vi "Update.vi"(8 "error in (no error)":errorcluster, 10 "Message in":refnum<class "UpdateMessage.lvclass">, 11 "Thorcam in":refnum<class "Thorcam.lvclass">) -> (0 "error out":errorcluster, 3 "Thorcam out":refnum<class "Thorcam.lvclass">)   [LabVIEW 2012, in "Thorcam.lvclass"]
doc: "The update method processes the command 'update'. \n\nThe command 'update' is used for receiving new values to be set to the private data of the class. This could be seen as a public set method for setting new parameters to the private class data."
uses:
  Thorcam.lvclass
  <vilib>/Distrio/Murmex/UpdateMessage/UpdateMessage.lvclass
  Thorcam.lvclass/Thorcam.ctl
  feed.ctl
  <vilib>/Distrio/Murmex/Murmex/Murmex.lvclass
panel:
  # "This method is called when the UPDATE\ntrigger is sent. \n\nOverride this method when your component needs to\nrespond to this trigger. \n\nCall parent for proper implementation"
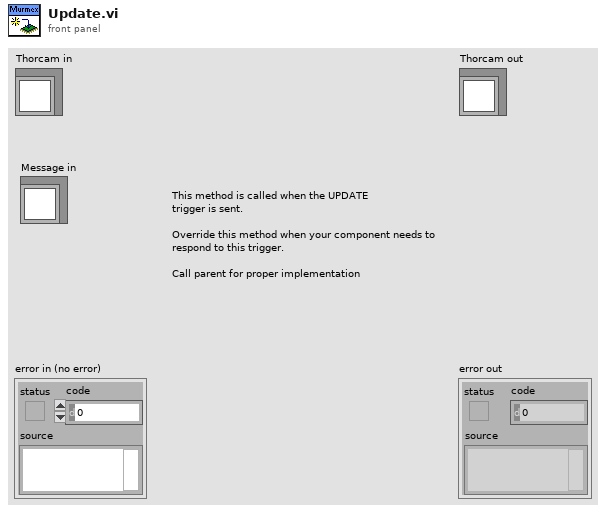
[diagram p1: front panel]
types:
  T1 = typedef "Thorcam.lvclass/feed.ctl" = enum16{"Video", "Cross Correlation", "Rob and Roy", "Roy", "Rob"}
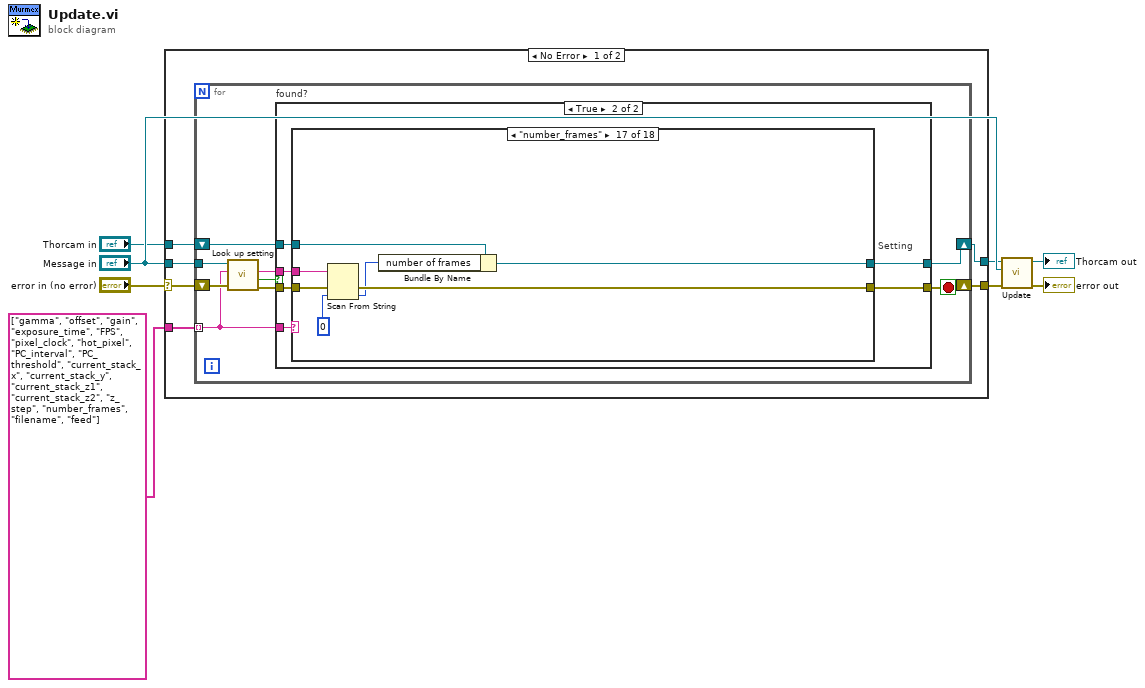
[diagram p0: block diagram]
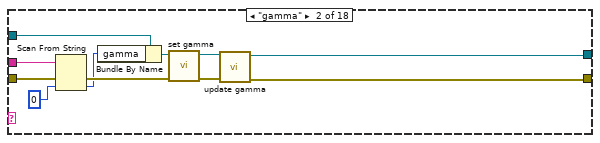
[diagram p4: hidden frame]
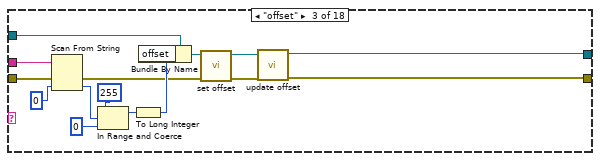
[diagram p5: hidden frame]
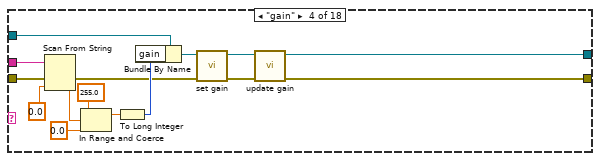
[diagram p6: hidden frame]
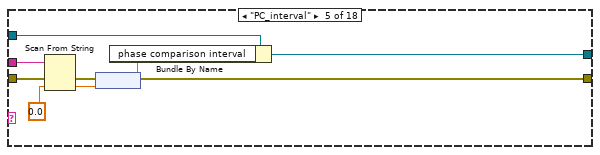
[diagram p7: hidden frame]
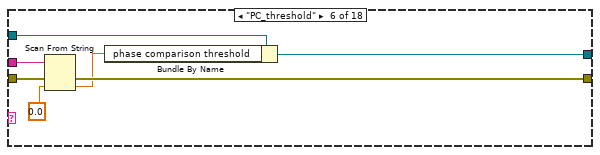
[diagram p8: hidden frame]
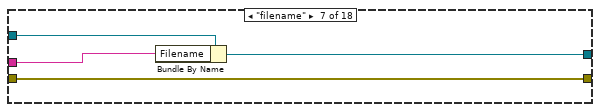
[diagram p9: hidden frame]
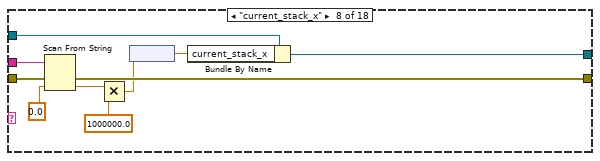
[diagram p10: hidden frame]
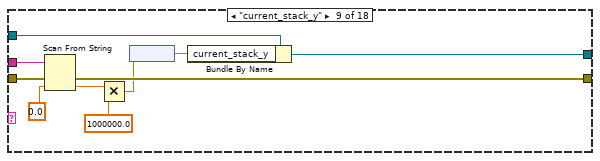
[diagram p11: hidden frame]
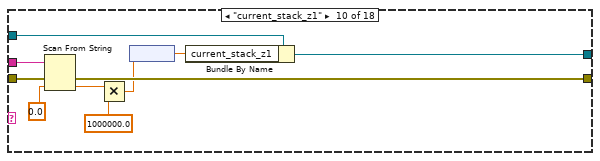
[diagram p12: hidden frame]
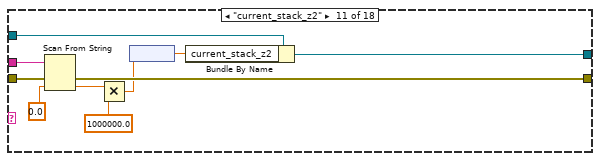
[diagram p13: hidden frame]
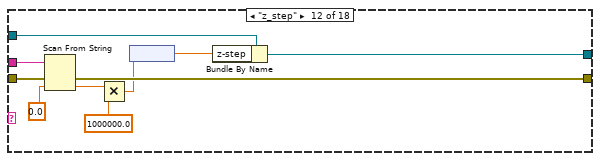
[diagram p14: hidden frame]
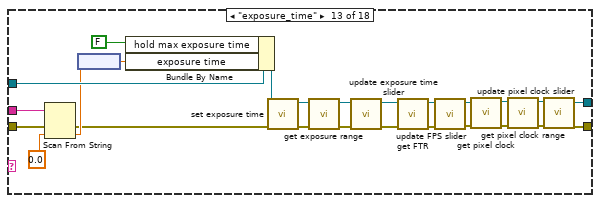
[diagram p15: hidden frame]
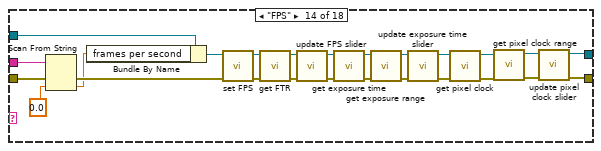
[diagram p16: hidden frame]
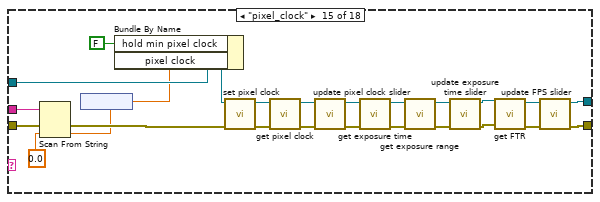
[diagram p17: hidden frame]
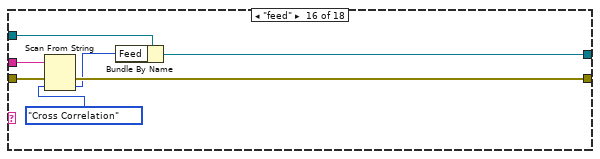
[diagram p18: hidden frame]
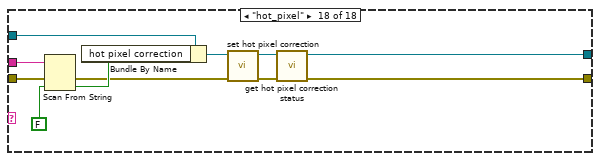
[diagram p19: hidden frame]
diagram:
  n1 = case shown="No Error" "error in (no error)" {
    selector: "error in (no error)" -> [w14 w245]
    tunnel: string[] ["gamma", "offset", "gain", "exposure_time", "FPS", "pixel_clock", "hot_pixel", "PC_interval", "PC_threshold", "current_stack_x", "current_stack_y", "current_stack_z1", "current_stack_z2", "z_step", "number_frames", "filename", "feed"] ("key chains") -> [w13 _]
    tunnel: "Message in" -> [w12 _]
    tunnel: "Thorcam in" -> [w11 w244]
    tunnel: [w10 w244] -> w2
    tunnel: [w9 w245] -> w1
    frame No Error {
      n2 = for {
        shift-right: [w16] -> w9
        shift-left: w14 -> [w23]
        tunnel: w13 -> [w21] mode=indexing
        tunnel: w12 -> [w20]
        shift-right: [w15] -> w10
        shift-left: w11 -> [w19]
        stop <- w16 stop-if-true
        n3 = call <vilib>:"Look up setting.vi"("error in (no error)"=w23, "tag name"=w21, "UpdateMessage in"=w20) -> ("error out"=w22:errorcluster, "found?"=w18:bool, "value"=w17:string)  [unwired: 5 in, 1 out]
        n4 = case "found?" shown="True" w18 {
          tunnel: w19 -> [w25 w30]
          tunnel: w17 -> [_ w31]
          tunnel: w22 -> [w24 w29]
          tunnel: w21 -> [_ w26]
          tunnel: [w25 w28] -> w15
          tunnel: [w24 w27] -> w16
          frame False {
          }
          frame True {
            n5 = case "Setting" shown="\"number_frames\"" w26 {
              tunnel: w31 -> [_ w43 w52 w73 w81 w88 w92 w102 w112 w122 w132 w142 w167 w192 w202 w224 w231 w242]
              tunnel: w30 -> [w33 w42 w59 w72 w80 w87 w93 w101 w111 w121 w131 w141 w166 w191 w218 w223 w230 w241]
              tunnel: w29 -> [w32 w44 w58 w74 w82 w89 w90 w103 w113 w123 w133 w143 w168 w193 w205 w225 w232 w243]
              tunnel: [w33 w35 w46 w60 w79 w86 w91 w100 w110 w120 w130 w140 w148 w174 w211 w222 w229 w233] -> w28
              tunnel: [w32 w34 w45 w61 w78 w85 w90 w99 w109 w119 w129 w139 w147 w170 w214 w221 w228 w236] -> w27
              frame Default {
              }
              frame "gamma" {
                n6 = Scan From String(input string=w43, error in=w44, default 1=0 ("settings.image.gamma")) -> (error out=w41:errorcluster, output 1=w39:i32)  [unwired: 2 in, 2 out]
                n7 = Bundle By Name(cluster=w42, "gamma"=w39) -> (w40:refnum<class "Thorcam.lvclass">)
                n8 = call-dynamic "set gamma.vi"("error in (no error)"=w41, "Thorcam in"=w40) -> ("error out"=w36:errorcluster, "Thorcam out"=w37:refnum<class "Thorcam.lvclass">)  [unwired: 8 in]
                n9 = call-dynamic "update gamma.vi"("error in (no error)"=w36, "Thorcam in"=w37) -> ("error out"=w34:errorcluster, "Thorcam out"=w35:refnum<class "Thorcam.lvclass">)  [unwired: 8 in]
              }
              frame "offset" {
                n10 = Scan From String(input string=w52, error in=w58, default 1=0 ("default value 1")) -> (error out=w51:errorcluster, output 1=w55:i32)  [unwired: 2 in, 2 out]
                n11 = In Range and Coerce(upper limit=255, x=w55, lower limit=0) -> (coerced(x)=w54:i32)  [unwired: 1 out]
                n12 = To Long Integer(number=w54) -> (32bit integer=w53:i32)
                n13 = Bundle By Name(cluster=w59, "offset"=w53) -> (w50:refnum<class "Thorcam.lvclass">)
                n14 = call-dynamic "set offset.vi"("error in (no error)"=w51, "Thorcam in"=w50) -> ("error out"=w47:errorcluster, "Thorcam out"=w48:refnum<class "Thorcam.lvclass">)  [unwired: 8 in]
                n15 = call-dynamic "update offset.vi"("error in (no error)"=w47, "Thorcam in"=w48) -> ("error out"=w45:errorcluster, "Thorcam out"=w46:refnum<class "Thorcam.lvclass">)  [unwired: 8 in]
              }
              frame "gain" {
                n16 = Scan From String(input string=w73, error in=w74, default 1=0.0 ("settings.Superactuator")) -> (error out=w65:errorcluster, output 1=w68:dbl)  [unwired: 2 in, 2 out]
                n17 = In Range and Coerce(upper limit=255.0, x=w68, lower limit=0.0) -> (coerced(x)=w66:dbl)  [unwired: 1 out]
                n18 = To Long Integer(number=w66) -> (32bit integer=w67:i32)
                n19 = Bundle By Name(cluster=w72, "gain"=w67) -> (w64:refnum<class "Thorcam.lvclass">)
                n20 = call-dynamic "set gain.vi"("error in (no error)"=w65, "Thorcam in"=w64) -> ("error out"=w62:errorcluster, "Thorcam out"=w63:refnum<class "Thorcam.lvclass">)  [unwired: 8 in]
                n21 = call-dynamic "update gain.vi"("error in (no error)"=w62, "Thorcam in"=w63) -> ("error out"=w61:errorcluster, "Thorcam out"=w60:refnum<class "Thorcam.lvclass">)  [unwired: 8 in]
              }
              frame "PC_interval" {
                n22 = Scan From String(input string=w81, error in=w82, default 1=0.0 ("settings.Superactuator")) -> (error out=w78:errorcluster, output 1=w76:dbl)  [unwired: 2 in, 2 out]
                n23 = node(w76) -> (w75:dbl[unit])
                n24 = Bundle By Name(cluster=w80, "phase comparison interval"=w75) -> (w79:refnum<class "Thorcam.lvclass">)
              }
              frame "PC_threshold" {
                n25 = Scan From String(input string=w88, error in=w89, default 1=0.0 ("settings.Superactuator")) -> (error out=w85:errorcluster, output 1=w83:dbl)  [unwired: 2 in, 2 out]
                n26 = Bundle By Name(cluster=w87, "phase comparison threshold"=w83) -> (w86:refnum<class "Thorcam.lvclass">)
              }
              frame "filename" {
                n27 = Bundle By Name(cluster=w93, "Filename"=w92) -> (w91:refnum<class "Thorcam.lvclass">)
              }
              frame "current_stack_x" {
                n28 = Scan From String(input string=w102, error in=w103, default 1=0.0 ("settings.Superactuator")) -> (error out=w99:errorcluster, output 1=w96:dbl)  [unwired: 2 in, 2 out]
                n29 = Multiply(x=w96, y=1000000.0) -> (x*y=w95:dbl)
                n30 = node(w95) -> (w94:dbl[unit])
                n31 = Bundle By Name(cluster=w101, "current_stack_x"=w94) -> (w100:refnum<class "Thorcam.lvclass">)
              }
              frame "current_stack_y" {
                n32 = Scan From String(input string=w112, error in=w113, default 1=0.0 ("settings.Superactuator")) -> (error out=w109:errorcluster, output 1=w106:dbl)  [unwired: 2 in, 2 out]
                n33 = Multiply(x=w106, y=1000000.0) -> (x*y=w105:dbl)
                n34 = node(w105) -> (w104:dbl[unit])
                n35 = Bundle By Name(cluster=w111, "current_stack_y"=w104) -> (w110:refnum<class "Thorcam.lvclass">)
              }
              frame "current_stack_z1" {
                n36 = Scan From String(input string=w122, error in=w123, default 1=0.0 ("settings.Superactuator")) -> (error out=w119:errorcluster, output 1=w116:dbl)  [unwired: 2 in, 2 out]
                n37 = Multiply(x=w116, y=1000000.0) -> (x*y=w115:dbl)
                n38 = node(w115) -> (w114:dbl[unit])
                n39 = Bundle By Name(cluster=w121, "current_stack_z1"=w114) -> (w120:refnum<class "Thorcam.lvclass">)
              }
              frame "current_stack_z2" {
                n40 = Scan From String(input string=w132, error in=w133, default 1=0.0 ("settings.Superactuator")) -> (error out=w129:errorcluster, output 1=w126:dbl)  [unwired: 2 in, 2 out]
                n41 = Multiply(x=w126, y=1000000.0) -> (x*y=w125:dbl)
                n42 = node(w125) -> (w124:dbl[unit])
                n43 = Bundle By Name(cluster=w131, "current_stack_z2"=w124) -> (w130:refnum<class "Thorcam.lvclass">)
              }
              frame "z_step" {
                n44 = Scan From String(input string=w142, error in=w143, default 1=0.0 ("settings.Superactuator")) -> (error out=w139:errorcluster, output 1=w136:dbl)  [unwired: 2 in, 2 out]
                n45 = Multiply(x=w136, y=1000000.0) -> (x*y=w135:dbl)
                n46 = node(w135) -> (w134:dbl[unit])
                n47 = Bundle By Name(cluster=w141, "z-step"=w134) -> (w140:refnum<class "Thorcam.lvclass">)
              }
              frame "exposure_time" {
                n48 = Scan From String(input string=w167, error in=w168, default 1=0.0 ("settings.Superactuator")) -> (error out=w160:errorcluster, output 1=w164:dbl)  [unwired: 2 in, 2 out]
                n49 = node(w164) -> (w163:dbl[unit])
                n50 = Bundle By Name(cluster=w166, "hold max exposure time"=FALSE ("runtime.exposure range.max exposure time"), "exposure time"=w163) -> (w159:refnum<class "Thorcam.lvclass">)
                n51 = call-dynamic "set exposure time.vi"("error in (no error)"=w160, "Thorcam in"=w159) -> ("error out"=w156:errorcluster, "Thorcam out"=w158:refnum<class "Thorcam.lvclass">)  [unwired: 8 in]
                n52 = call-dynamic "get exposure range.vi"("error in (no error)"=w156, "Thorcam in"=w158) -> ("error out"=w155:errorcluster, "Thorcam out"=w157:refnum<class "Thorcam.lvclass">)  [unwired: 8 in]
                n53 = call-dynamic "update exposure time slider.vi"("error in (no error)"=w155, "Thorcam in"=w157) -> ("error out"=w145:errorcluster, "Thorcam out"=w146:refnum<class "Thorcam.lvclass">)  [unwired: 8 in]
                n54 = call-dynamic "get FTR.vi"("error in (no error)"=w145, "Thorcam in"=w146) -> ("error out"=w162:errorcluster, "Thorcam out"=w161:refnum<class "Thorcam.lvclass">)  [unwired: 8 in]
                n55 = call-dynamic "update FPS slider.vi"("error in (no error)"=w162, "Thorcam in"=w161) -> ("error out"=w154:errorcluster, "Thorcam out"=w153:refnum<class "Thorcam.lvclass">)  [unwired: 8 in]
                n56 = call-dynamic "get pixel clock.vi"("error in (no error)"=w154, "Thorcam in"=w153) -> ("error out"=w151:errorcluster, "Thorcam out"=w152:refnum<class "Thorcam.lvclass">)  [unwired: 8 in]
                n57 = call-dynamic "get pixel clock range.vi"("error in (no error)"=w151, "Thorcam in"=w152) -> ("error out"=w149:errorcluster, "Thorcam out"=w150:refnum<class "Thorcam.lvclass">)  [unwired: 8 in]
                n58 = call-dynamic "update pixel clock slider.vi"("error in (no error)"=w149, "Thorcam in"=w150) -> ("error out"=w147:errorcluster, "Thorcam out"=w148:refnum<class "Thorcam.lvclass">)  [unwired: 8 in]
              }
              frame "FPS" {
                n59 = Scan From String(input string=w192, error in=w193, default 1=0.0 ("settings.Superactuator")) -> (error out=w187:errorcluster, output 1=w169:dbl)  [unwired: 2 in, 2 out]
                n60 = Bundle By Name(cluster=w191, "frames per second"=w169) -> (w186:refnum<class "Thorcam.lvclass">)
                n61 = call-dynamic "set FPS.vi"("error in (no error)"=w187, "Thorcam in"=w186) -> ("error out"=w184:errorcluster, "Thorcam out"=w185:refnum<class "Thorcam.lvclass">)  [unwired: 8 in]
                n62 = call-dynamic "get FTR.vi"("error in (no error)"=w184, "Thorcam in"=w185) -> ("error out"=w182:errorcluster, "Thorcam out"=w183:refnum<class "Thorcam.lvclass">)  [unwired: 8 in]
                n63 = call-dynamic "update FPS slider.vi"("error in (no error)"=w182, "Thorcam in"=w183) -> ("error out"=w179:errorcluster, "Thorcam out"=w181:refnum<class "Thorcam.lvclass">)  [unwired: 8 in]
                n64 = call-dynamic "get exposure time.vi"("error in (no error)"=w179, "Thorcam in"=w181) -> ("error out"=w178:errorcluster, "Thorcam out"=w180:refnum<class "Thorcam.lvclass">)  [unwired: 7 in, 1 out]
                n65 = call-dynamic "get exposure range.vi"("error in (no error)"=w178, "Thorcam in"=w180) -> ("error out"=w189:errorcluster, "Thorcam out"=w188:refnum<class "Thorcam.lvclass">)  [unwired: 8 in]
                n66 = call-dynamic "update exposure time slider.vi"("error in (no error)"=w189, "Thorcam in"=w188) -> ("error out"=w173:errorcluster, "Thorcam out"=w177:refnum<class "Thorcam.lvclass">)  [unwired: 8 in]
                n67 = call-dynamic "get pixel clock.vi"("error in (no error)"=w173, "Thorcam in"=w177) -> ("error out"=w172:errorcluster, "Thorcam out"=w176:refnum<class "Thorcam.lvclass">)  [unwired: 8 in]
                n68 = call-dynamic "get pixel clock range.vi"("error in (no error)"=w172, "Thorcam in"=w176) -> ("error out"=w171:errorcluster, "Thorcam out"=w175:refnum<class "Thorcam.lvclass">)  [unwired: 8 in]
                n69 = call-dynamic "update pixel clock slider.vi"("error in (no error)"=w171, "Thorcam in"=w175) -> ("error out"=w170:errorcluster, "Thorcam out"=w174:refnum<class "Thorcam.lvclass">)  [unwired: 8 in]
              }
              frame "pixel_clock" {
                n70 = Scan From String(input string=w202, error in=w205, default 1=0.0 ("settings.Superactuator")) -> (error out=w204:errorcluster, output 1=w203:dbl)  [unwired: 2 in, 2 out]
                n71 = node(w203) -> (w217:dbl[unit])
                n72 = Bundle By Name(cluster=w218, "hold min pixel clock"=FALSE ("runtime.pixel clock range.hold minimum"), "pixel clock"=w217) -> (w210:refnum<class "Thorcam.lvclass">)
                n73 = call-dynamic "set pixel clock.vi"("error in (no error)"=w204, "Thorcam in"=w210) -> ("error out"=w196:errorcluster, "Thorcam out"=w198:refnum<class "Thorcam.lvclass">)  [unwired: 8 in]
                n74 = call-dynamic "get pixel clock.vi"("error in (no error)"=w196, "Thorcam in"=w198) -> ("error out"=w195:errorcluster, "Thorcam out"=w197:refnum<class "Thorcam.lvclass">)  [unwired: 8 in]
                n75 = call-dynamic "update pixel clock slider.vi"("error in (no error)"=w195, "Thorcam in"=w197) -> ("error out"=w208:errorcluster, "Thorcam out"=w209:refnum<class "Thorcam.lvclass">)  [unwired: 8 in]
                n76 = call-dynamic "get exposure time.vi"("error in (no error)"=w208, "Thorcam in"=w209) -> ("error out"=w207:errorcluster, "Thorcam out"=w206:refnum<class "Thorcam.lvclass">)  [unwired: 7 in, 1 out]
                n77 = call-dynamic "get exposure range.vi"("error in (no error)"=w207, "Thorcam in"=w206) -> ("error out"=w216:errorcluster, "Thorcam out"=w213:refnum<class "Thorcam.lvclass">)  [unwired: 8 in]
                n78 = call-dynamic "update exposure time slider.vi"("error in (no error)"=w216, "Thorcam in"=w213) -> ("error out"=w199:errorcluster, "Thorcam out"=w200:refnum<class "Thorcam.lvclass">)  [unwired: 8 in]
                n79 = call-dynamic "get FTR.vi"("error in (no error)"=w199, "Thorcam in"=w200) -> ("error out"=w215:errorcluster, "Thorcam out"=w212:refnum<class "Thorcam.lvclass">)  [unwired: 8 in]
                n80 = call-dynamic "update FPS slider.vi"("error in (no error)"=w215, "Thorcam in"=w212) -> ("error out"=w214:errorcluster, "Thorcam out"=w211:refnum<class "Thorcam.lvclass">)  [unwired: 8 in]
              }
              frame "feed" {
                n81 = Scan From String(input string=w224, error in=w225, default 1=feed."Cross Correlation" ("settings.Feed")) -> (error out=w221:errorcluster, output 1=w220:T1)  [unwired: 2 in, 2 out]
                n82 = Bundle By Name(cluster=w223, "Feed"=w220) -> (w222:refnum<class "Thorcam.lvclass">)
              }
              frame "number_frames" {
                n83 = Scan From String(input string=w231, error in=w232, default 1=0 ("settings.trigger.trigger edge")) -> (error out=w228:errorcluster, output 1=w226:i32)  [unwired: 2 in, 2 out]
                n84 = Bundle By Name(cluster=w230, "number of frames"=w226) -> (w229:refnum<class "Thorcam.lvclass">)
              }
              frame "hot_pixel" {
                n85 = Scan From String(input string=w242, error in=w243, default 1=FALSE ("settings.image.hot pixel correction")) -> (error out=w237:errorcluster, output 1=w239:bool)  [unwired: 2 in, 2 out]
                n86 = Bundle By Name(cluster=w241, "hot pixel correction"=w239) -> (w234:refnum<class "Thorcam.lvclass">)
                n87 = call-dynamic "set hot pixel correction.vi"("error in (no error)"=w237, "Thorcam in"=w234) -> ("error out"=w238:errorcluster, "Thorcam out"=w235:refnum<class "Thorcam.lvclass">)  [unwired: 8 in]
                n88 = call-dynamic "get hot pixel correction status.vi"("error in (no error)"=w238, "Thorcam in"=w235) -> ("error out"=w236:errorcluster, "Thorcam out"=w233:refnum<class "Thorcam.lvclass">)  [unwired: 8 in]
              }
            }
          }
        }
      }
    }
    frame Error {
    }
  }
  n89 = call-parent "Update.vi"("error in (no error)"=w1, "Message in"="Message in", "Murmex in"=w2) -> ("error out"=→"error out":errorcluster, "Murmex out"=→"Thorcam out":refnum<class "Thorcam.lvclass">)  [unwired: 7 in]
